vi "Receive UI Command.vi"(10 "Consumer Queues in":T1) -> (0 "error out":errorcluster, 2 "Consumer Queues out":T1, 3 "UI Process Command out":refnum<class "Generic UI Process Command.lvclass">)   [LabVIEW 2019, in "User Interface Process.lvlib" / "Generic UI Process Command.lvclass"]
uses:
  Generic UI Process Command.lvclass
  TS Framework/Consumer Queues.ctl
  DAC Process/Generic DAC Command/Generic DAC Process Command.lvclass
  Trig Process/Generic Trig Command/Generic Trig Process Command.lvclass
  TS Framework/TS Framework.lvlib
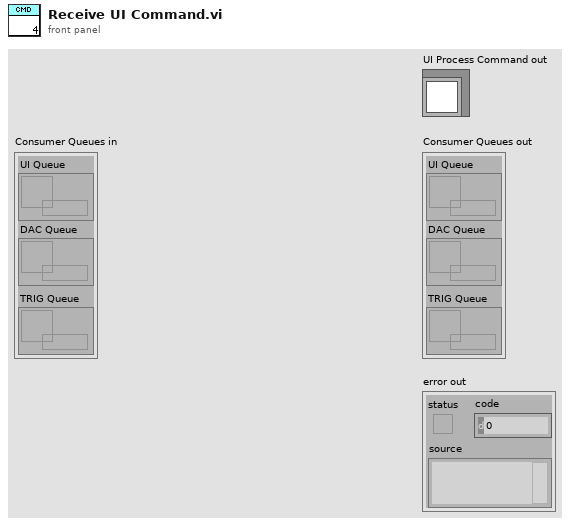
[diagram p1: front panel]
types:
  T1 = typedef "TS Framework.lvlib/Consumer Queues.ctl" = cluster{"UI Queue":refnum<queue>, "DAC Queue":refnum<queue>, "TRIG Queue":refnum<queue>}
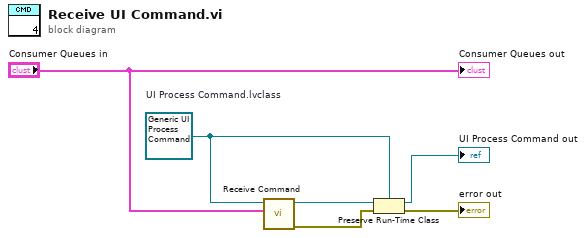
[diagram p0: block diagram]
diagram:
  w3 = refnum<class "Generic UI Process Command.lvclass"> refnum  # UI Process Command.lvclass
  n1 = call-dynamic "Receive Command.vi"("Consumer Queues"="Consumer Queues in", "UI Process Command in"=w3) -> ("error out"=w5:errorcluster, "Generic Command out"=w4:refnum<class "Generic Command.lvclass">)  [unwired: 8 in]
  n2 = Preserve Run-Time Class(object in=w4, error in=w5, 2:w3) -> (object out=→"UI Process Command out":refnum<class "Generic UI Process Command.lvclass">, error out=→"error out":errorcluster)
  "Consumer Queues out" <- "Consumer Queues in"
